vi "SetRemote.vi"(6 "Remote?":bool, 8 "ErrorIn":errorcluster, 9 "ServiceName":string, 10 "MachineName":string, 11 "YActorIn":refnum<class "YActor.lvclass">) -> (0 "ErrorOut":errorcluster, 3 "YActorOut":refnum<class "YActor.lvclass">)   [LabVIEW 2021, in "YActor.lvclass"]
uses:
  YActor.lvclass
  YActor.lvclass/YActor.ctl
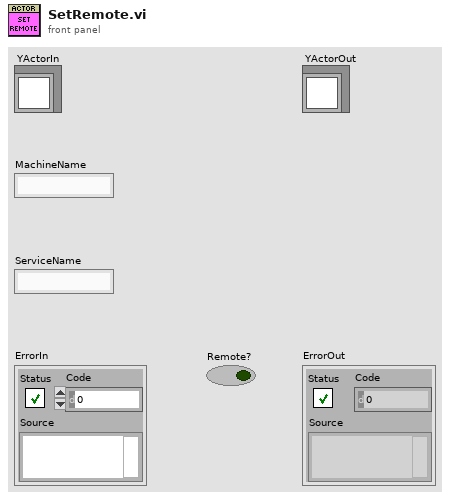
[diagram p1: front panel]
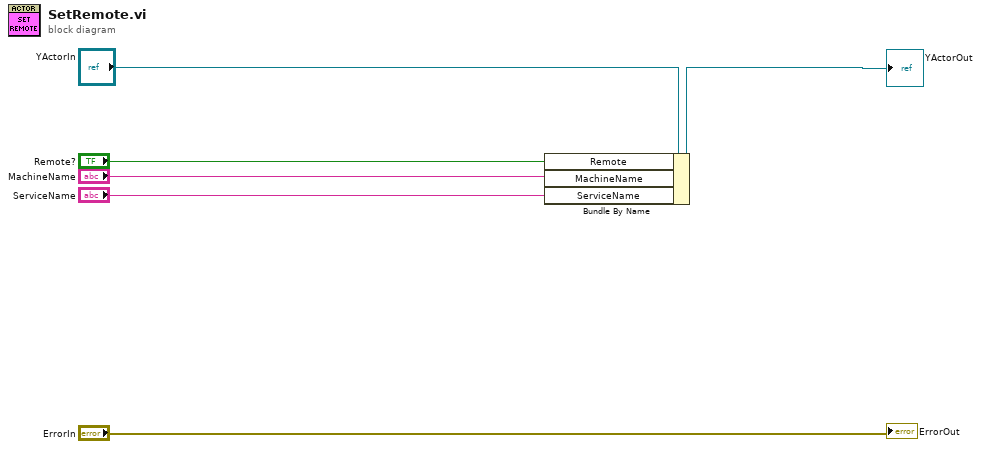
[diagram p0: block diagram]
diagram:
  n1 = Bundle By Name(cluster="YActorIn", "Remote"="Remote?", "MachineName"="MachineName", "ServiceName"="ServiceName") -> (→"YActorOut":refnum<class "YActor.lvclass">)
  "ErrorOut" <- "ErrorIn"
